vi "FlpLib IIRDirectFormIITrans1stOrder 4.vi"(0 "xn":sgl, 1 "ak":sgl, 2 "bk":sgl, 11 "stateIn":sgl) -> (4 "yn":sgl, 15 "stateOut":sgl)   [LabVIEW 2017]
uses:
  <userlib>/_NI FLP Library/FPGA/outsideSCTL/FlpLib Multiply Shared Instance 4.vi
  <userlib>/_NI FLP Library/FPGA/outsideSCTL/FlpLib Add Shared Instance 4.vi
  <userlib>/_NI FLP Library/FPGA/outsideSCTL/FlpLib Subtract Shared Instance 4.vi
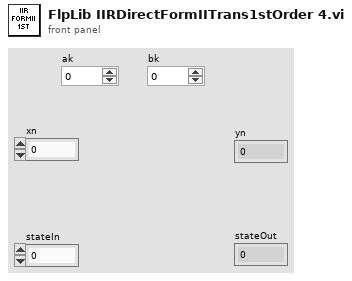
[diagram p1: front panel]
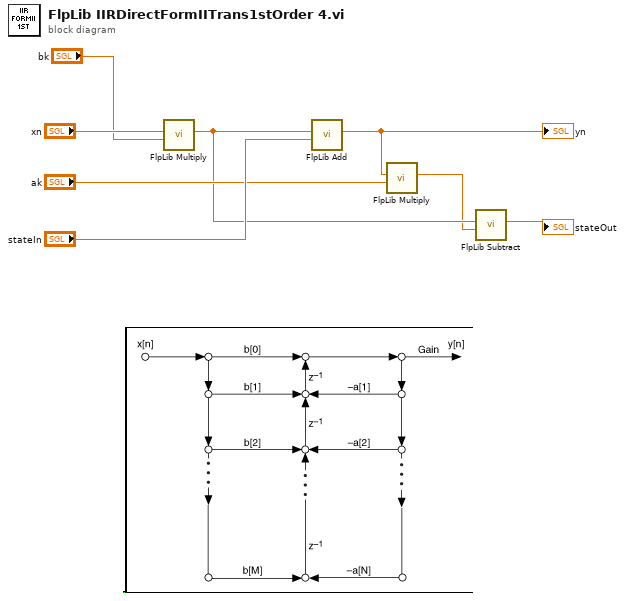
[diagram p0: block diagram]
diagram:
  n1 = call-poly <userlib>:"FlpLib Multiply.vi"("y"="bk", "x"="xn") -> ("x*y"=w3:sgl)  [unwired: 5 in]
  n2 = call-poly <userlib>:"FlpLib Add.vi"("y"="stateIn", "x"=w3) -> ("x+y"=w5:sgl)  [unwired: 5 in]
  "yn" <- w5
  n3 = call-poly <userlib>:"FlpLib Multiply.vi"("y"="ak", "x"=w5) -> ("x*y"=w1:sgl)  [unwired: 5 in]
  n4 = call-poly <userlib>:"FlpLib Subtract.vi"("y"=w1, "x"=w3) -> ("x-y"=→"stateOut":sgl)  [unwired: 5 in]
